vi "Extract boolean parameter.vi"(8 "error in (no error)":errorcluster, 9 "parameter":string, 10 "Message in":refnum<class "GenericMessage.lvclass">, 11 "Tomo in":refnum<class "Tomo.lvclass">) -> (0 "error out":errorcluster, 2 "parameter":bool, 3 "Tomo out":refnum<class "Tomo.lvclass">)   [LabVIEW 2012, in "Tomo.lvclass"]
uses:
  Tomo.lvclass
  <vilib>/Distrio/Murmex/GenericMessage/GenericMessage.lvclass
  <vilib>/Distrio/Murmex/Message/Message.lvclass
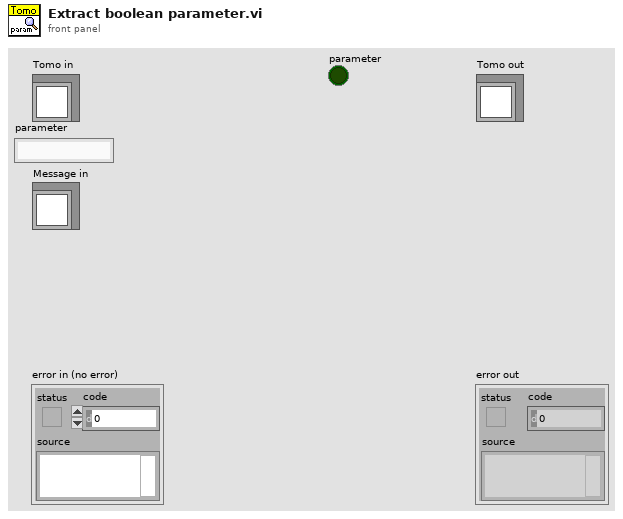
[diagram p1: front panel]
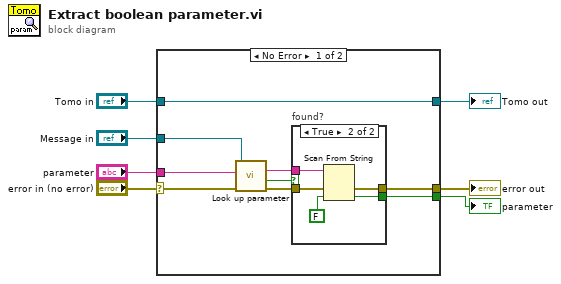
[diagram p0: block diagram]
diagram:
  n1 = case shown="No Error" "error in (no error)" {
    selector: "error in (no error)" -> [w12 w24]
    tunnel: [w11 w24] -> w6
    tunnel: [w16 w23] -> w4
    tunnel: "Tomo in" -> [w16 w23]
    tunnel: "Message in" -> [w10 _]
    tunnel: [w9 _] -> w2
    tunnel: "parameter" -> [w8 _]
    frame No Error {
      n2 = call <vilib>:"Look up parameter.vi"("error in (no error)"=w12, "name"=w8, "Message in"=w10) -> ("error out"=w15:errorcluster, "found?"=w13:bool, "key"=w14:string)  [unwired: 5 in, 1 out]
      n3 = case "found?" shown="True" w13 {
        tunnel: w15 -> [w17 w21]
        tunnel: w14 -> [_ w20]
        tunnel: [w17 w19] -> w11
        tunnel: [_ w18] -> w9
        frame False {
        }
        frame True {
          n4 = Scan From String(input string=w20, error in=w21, default 1=FALSE) -> (error out=w19:errorcluster, output 1=w18:bool)  [unwired: 2 in, 2 out]
        }
      }
    }
    frame Error {
    }
  }
  "error out" <- w6
  "Tomo out" <- w4
  "parameter" <- w2
